vi "Duplicate.vi"(8 "error in":errorcluster, 10 "parameters":variant, 11 "PS Instrument":refnum<class "Power Supply Instrument.lvclass">) -> (0 "error out":errorcluster, 3 "PS Instrument out":refnum<class "Power Supply Instrument.lvclass">)   [LabVIEW 2025, in "Power Supply.lvlib" / "Power Supply Instrument.lvclass"]
doc: "Implements the specific behavior of a node when it is being duplicated\nCan be used to change the name of the new node for example adding Copy to it. \nCopyright 2017 National Instruments Corporation\n\nLicensed under the Apache License, Version 2.0 (the \"License\"); you may not use this file except in compliance with the License. You may obtain a copy of the License at http://www.apache.org/licenses/LICENSE-2.0\nUnless required by applicable law or agreed to in writing, software distributed under the License is distributed on an \"AS IS\" BASIS, WITHOUT WARRANTIES OR CONDITIONS OF ANY KIND, either express or implied. See the License for the specific language governing permissions and limitations under the License."
uses:
  Power Supply Instrument.lvclass
  Power Supply Instrument.lvclass/Power Supply Instrument.ctl
  Users/Public/Documents/Sandia National Labs/TSS Plugin/Abstract Engine.lvlibp/Plugin/Abstract/Instrument configuration/Instrument configuration.lvclass
  Users/Public/Documents/Sandia National Labs/TSS Plugin/Abstract Engine.lvlibp/Plugin/Abstract/Abstract Instrument/Abstract Instrument.lvclass
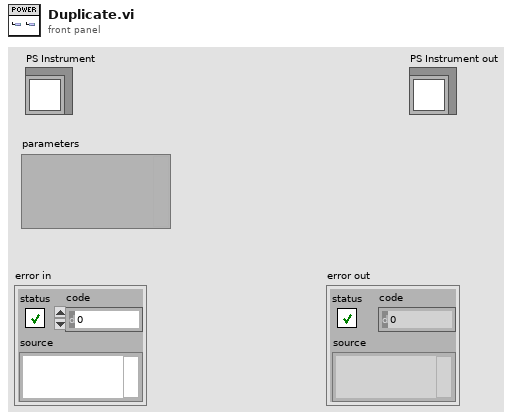
[diagram p1: front panel]
types:
  T1 = cluster{"Type":string, "Address":string, "SW Alias":string, "Description":string, "Enabled":bool}
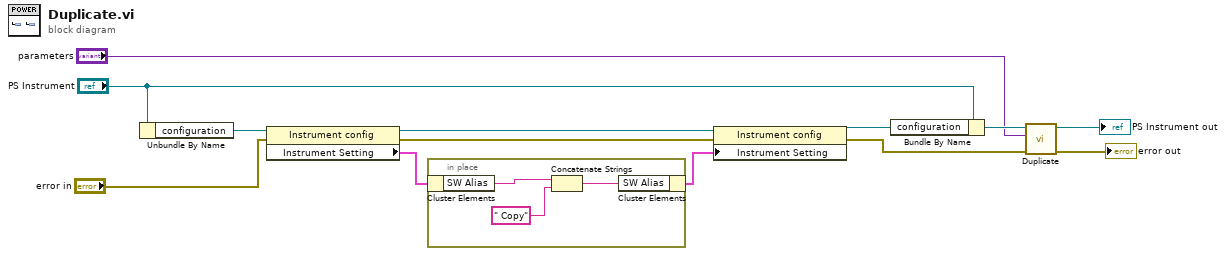
[diagram p0: block diagram]
diagram:
  n1 = Unbundle By Name("PS Instrument") -> ("configuration"=w7:refnum<class "Instrument configuration.lvclass">)
  n2 = property class="Instrument config"(reference=w7, error in="error in") -> (reference out=w4:refnum<class "Instrument configuration.lvclass">, error out=w5:errorcluster, "Instrument Setting"=w3:T1)
  n3 = in-place {
    n4 = in-place-cluster #1(w3) -> ("SW Alias"=w16:string)
    n5 = Concatenate Strings(w16, " Copy") -> (w15:string)
    n6 = in-place-cluster #1("SW Alias"=w15) -> (w1:T1)
  }
  n7 = property class="Instrument config"(reference=w4, error in=w5, "Instrument Setting"=w1) -> (reference out=w6:refnum<class "Instrument configuration.lvclass">, error out=w10:errorcluster)
  n8 = Bundle By Name(cluster="PS Instrument", "configuration"=w6) -> (w12:refnum<class "Power Supply Instrument.lvclass">)
  n9 = call-parent "Duplicate.vi"("error in"=w10, "parameters"="parameters", "CEF_Serialize node in"=w12) -> ("error out"=→"error out":errorcluster, "CEF_Serialize node out"=→"PS Instrument out":refnum<class "Power Supply Instrument.lvclass">)  [unwired: 7 in]
